vi "Start.vi"(8 "error in (no error)":errorcluster caption="entrée d'erreur (pas d'erreur)", 11 "DAQmxTaskContainer en entrée":refnum<class "DAQmxTaskContainer.lvclass">) -> (0 "error out":errorcluster caption="sortie d'erreur", 3 "DAQmxTaskContainer en sortie":refnum<class "DAQmxTaskContainer.lvclass">)   [LabVIEW 2015, in "DAQmxTaskContainer.lvclass"]
uses:
  DAQmxTaskContainer.lvclass
  dependecies/ControlsVIs/Clusters-def/SERVER-Commands.ctl
  dependecies/ControlsVIs/Clusters-def/Message types.ctl
  DAQmxTaskContainer.lvclass/DAQmxTaskContainer.ctl
  DAQmxTask.lvclass
  Message/Message.lvclass
  Control/Control-Server/Control-Server.lvclass
  GeneralFunctionality/GeneralFunctionality.lvclass
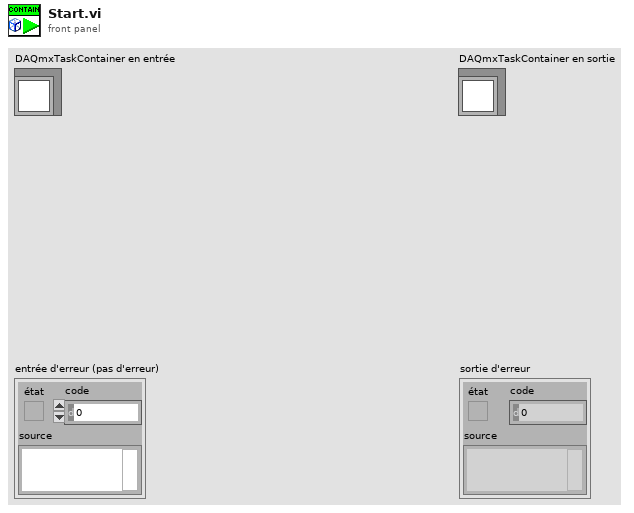
[diagram p1: front panel]
types:
  T1 = typedef "Message types.ctl" = string
  T2 = typedef "Control-Server.lvclass/SERVER-Commands.ctl" = string
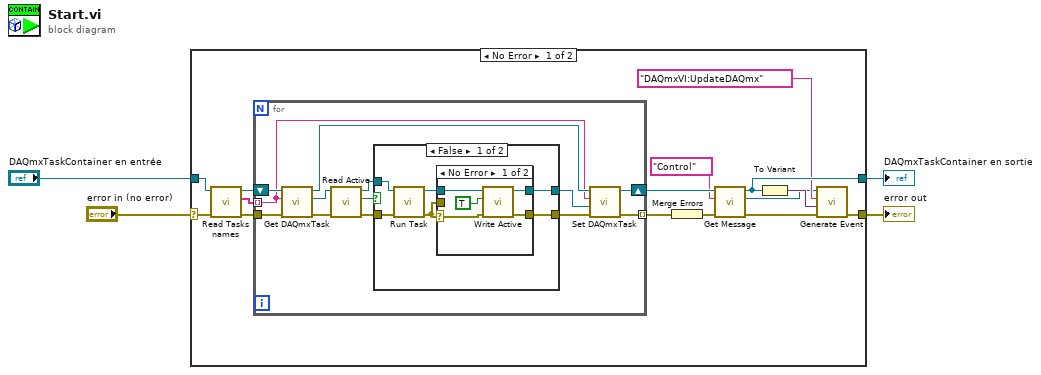
[diagram p0: block diagram]
diagram:
  n1 = case shown="No Error" "error in (no error)" {
    selector: "error in (no error)" -> [w10 w49]
    tunnel: [w15 w49] -> w3
    tunnel: [w17 w48] -> w1
    tunnel: "DAQmxTaskContainer en entrée" -> [w7 w48]
    frame No Error {
      n2 = call "Read Tasks names.vi"("error in (no error)"=w10, "DAQmxTaskContainer en entrée"=w7) -> ("error out"=w9:errorcluster, "Tasks names"=w6:string[], "DAQmxTaskContainer en sortie"=w8:refnum<class "DAQmxTaskContainer.lvclass">)  [unwired: 7 in]
      n3 = for {
        tunnel: w6 -> [w24] mode=indexing
        tunnel: w9 -> [w28]
        tunnel: [w23] -> w19 mode=indexing
        shift-right: [w21] -> w16
        shift-left: w8 -> [w29]
        n4 = call "Get DAQmxTask.vi"("error in (no error)"=w28, "Task name"=w24, "DAQmxTaskContainer in"=w29) -> ("error out"=w26:errorcluster, "DAQmx Task"=w27:refnum<class "DAQmxTask.lvclass">, "DAQmxTaskContainer out"=w25:refnum<class "DAQmxTaskContainer.lvclass">)  [unwired: 6 in]
        n5 = call-dynamic "Read Active.vi"("error in (no error)"=w26, "DAQmxTask in"=w27) -> ("error out"=w30:errorcluster, "Active?"=w32:bool, "DAQmxTask out"=w31:refnum<class "DAQmxTask.lvclass">)  [unwired: 7 in]
        n6 = case shown="False" w32 {
          tunnel: w31 -> [w38 w47]
          tunnel: w30 -> [w37 w46]
          tunnel: [w36 w46] -> w22
          tunnel: [w35 w47] -> w20
          frame False {
            n7 = call "Run Task.vi"("error in (no error)"=w37, "DAQmxTask in"=w38) -> ("error out"=w33:errorcluster, "DAQmxTask out"=w34:refnum<class "DAQmxTask.lvclass">)  [unwired: 8 in]
            n8 = case shown="No Error" w33 {
              selector: w33 -> [w43 _]
              tunnel: [w41 w44] -> w36
              tunnel: [w40 w45] -> w35
              tunnel: w34 -> [w39 w45]
              tunnel: w33 -> [_ w44]
              frame No Error {
                n9 = call-dynamic "Write Active.vi"("error in (no error)"=w43, "Active?"=TRUE, "DAQmxTask in"=w39) -> ("error out"=w41:errorcluster, "DAQmxTask out"=w40:refnum<class "DAQmxTask.lvclass">)  [unwired: 7 in]
              }
              frame Error {
              }
            }
          }
          frame True {
          }
        }
        n10 = call "Set DAQmxTask.vi"("error in (no error)"=w22, "DAQmxTask"=w20, "Task name"=w24, "DAQmxTaskContainer in"=w25) -> ("error out"=w23:errorcluster, "DAQmxTaskContainer out"=w21:refnum<class "DAQmxTaskContainer.lvclass">)  [unwired: 6 in]
      }
      n11 = Merge Errors(w19) -> (w18:errorcluster)
      n12 = call "Get Message.vi"("error in (no error)"=w18, "Message type"=T1 "Control", "GeneralFunctionality en entrée"=w16) -> ("error out"=w11:errorcluster, "Message.lvclass"=w12:refnum<class "Message.lvclass">, "GeneralFunctionality en sortie"=w17:refnum<class "DAQmxTaskContainer.lvclass">)  [unwired: 6 in]
      n13 = To Variant(anything=w17) -> (Variant=w13:variant)
      n14 = call "Generate Event.vi"("error in (no error)"=w11, "Data"=w13, "Command"=T2 "DAQmxVI:UpdateDAQmx", "Message en entrée"=w12) -> ("error out"=w15:errorcluster)  [unwired: 6 in, 1 out]
    }
    frame Error {
    }
  }
  "error out" <- w3
  "DAQmxTaskContainer en sortie" <- w1
